vi "MatchPattern.vi"(10 "正则表达式":string, 11 "字符串":string="ÿÿÿÿÿÿÿÿÿÿÿÿÿÿÿÿÿÿÿÿÿÿÿÿÿÿÿ") -> (0 "Match":bool, 1 "匹配后偏移量":i32, 2 "HexStr":string, 3 "String":string)   [LabVIEW 2013]
panel:
  out "连接的字符串":string
  in  "Data":string=". \u0002\u0001\u0000Ü"
  in  "DataType":string=". \u0002\u0001\u0000Ü"
  out "子字符串之后":string
  out "匹配后偏移量 3":i32
  out "字符串 2":string
  out "offset past match":i32 caption="匹配后偏移量"
  out "result string":string caption="结果字符串"
  out "标记索引":i32
  out "标记字符串":string
  out "标记后偏移量":i32
  out "字符串输出":string
  out "正则表达式 3":string
  in  "正则表达式 2":string
  out "匹配偏移量":i32
  out "匹配+剩余字符串":string
  out "替换数量":i32
  out "结果字符串":string
  out "匹配后偏移量 2":i32
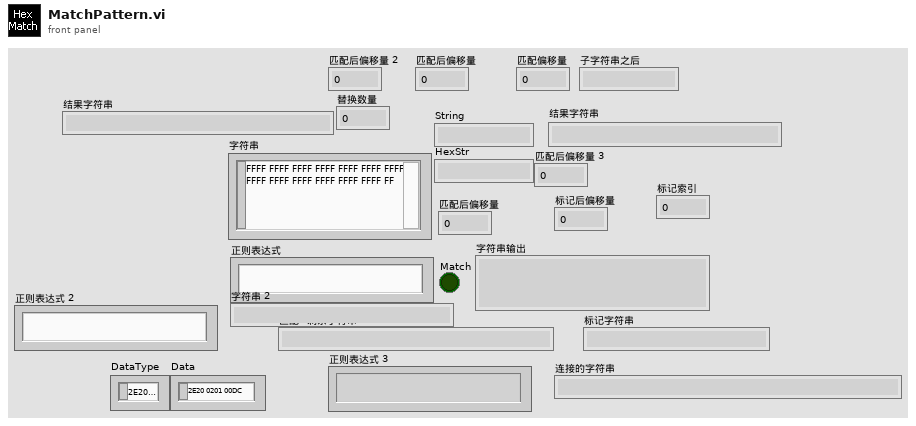
[diagram p1: front panel]
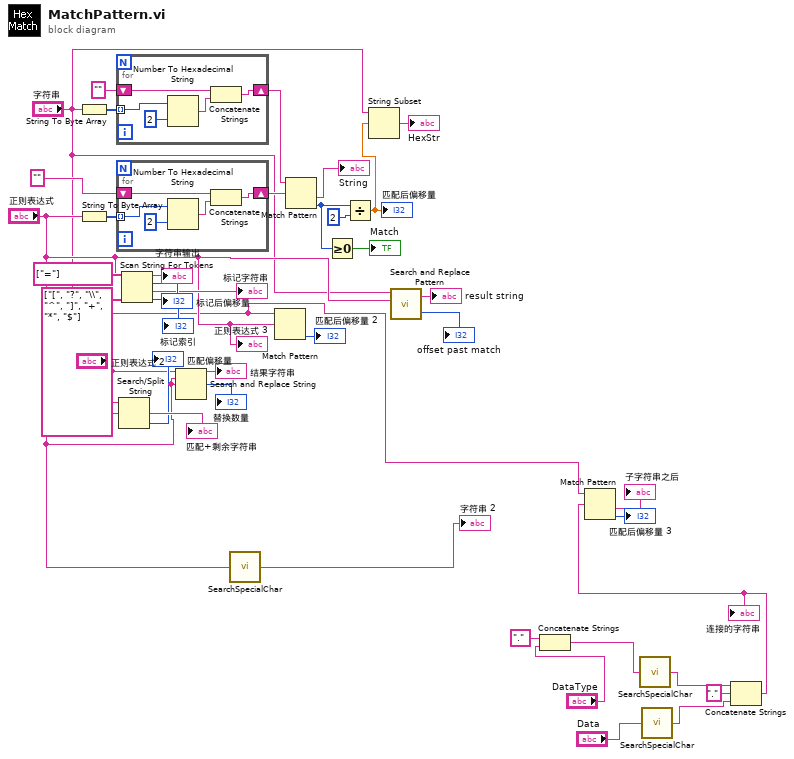
[diagram p0: block diagram]
diagram:
  n1 = String To Byte Array(string="字符串") -> (unsigned byte array=w38:u8[])
  n2 = String To Byte Array(string="正则表达式") -> (unsigned byte array=w34:u8[])
  n3 = for {
    shift-right: [w42] -> w36
    shift-left: "" -> [w41]
    tunnel: w38 -> [w39] mode=indexing
    n4 = Number To Hexadecimal String(1:i16 2 ("宽度(-)"), 2:w39) -> (0:w43:string)
    n5 = Concatenate Strings(w41, w43) -> (w42:string)
  }
  n6 = for {
    shift-right: [w47] -> w33
    shift-left: "" -> [w46]
    tunnel: w34 -> [w44] mode=indexing
    n7 = Number To Hexadecimal String(1:i16 2 ("宽度(-)"), 2:w44) -> (0:w48:string)
    n8 = Concatenate Strings(w46, w48) -> (w47:string)
  }
  n9 = Search/Split String(string="字符串", search string/char (-)="正则表达式") -> (match + rest of string=→"匹配+剩余字符串":string, offset of match=→"匹配偏移量":i32)  [unwired: 1 in, 1 out]
  n10 = Scan String For Tokens(6:string[] ["[", "?", "\\", "^", "]", "+", "*", "$"] ("分隔符(\\s,\\t,\\r,\\n)"), 7:string[] ["="] ("运算符（无）"), 9:"正则表达式") -> (0:→"标记索引":i32, 1:→"标记字符串":string, 2:→"标记后偏移量":i32, 3:→"字符串输出":string)  [unwired: 3 in]
  n11 = Search and Replace String(input string="字符串", search string="正则表达式", replace string="正则表达式") -> (result string=→"结果字符串":string, number of replacements=→"替换数量":i32)  [unwired: 5 in, 2 out]
  n12 = call "SearchSpecialChar.vi"("正则表达式"="正则表达式") -> ("字符串"=→"字符串 2":string)
  n13 = Match Pattern(string="字符串", regular expression="正则表达式") -> (offset past match=→"匹配后偏移量 2":i32)  [unwired: 1 in, 3 out]
  n14 = Match Pattern(string=w36, regular expression=w33) -> (after substring=→"String":string, offset past match=w31:i32)  [unwired: 1 in, 2 out]
  n15 = Greater Or Equal To 0?(x=w31) -> (x >= 0?=→"Match":bool)
  n16 = Divide(x=w31, y=2) -> (x/y=w28:dbl)
  "匹配后偏移量" <- w28
  n17 = String Subset(string="字符串", offset (0)=w28) -> (substring=→"HexStr":string)  [unwired: 1 in]
  n18 = call <vilib>:"Search and Replace Pattern.vi"("string"="字符串", "regular expression (\"\")"="正则表达式") -> ("result string"=→"result string":string, "offset past match"=→"offset past match":i32)  [unwired: 3 in]
  n19 = Concatenate Strings("." ("字符串"), "DataType") -> (w7:string)
  n20 = call "SearchSpecialChar.vi"("正则表达式"=w7) -> ("字符串"=w6:string)
  n21 = call "SearchSpecialChar.vi"("正则表达式"="Data") -> ("字符串"=w5:string)
  n22 = Concatenate Strings(w6, "." ("字符串"), w5) -> (w3:string)
  "连接的字符串" <- w3
  n23 = Match Pattern(string="字符串", regular expression=w3) -> (after substring=→"子字符串之后":string, offset past match=→"匹配后偏移量 3":i32)  [unwired: 1 in, 2 out]
  "正则表达式 3" <- "正则表达式"
